vi "mainVI.vi"() -> ()   [LabVIEW 2019]
panel:
  out "Waveform Graph":dbl[][](graph)
  in  "New plot":bool
  in  "stop":bool
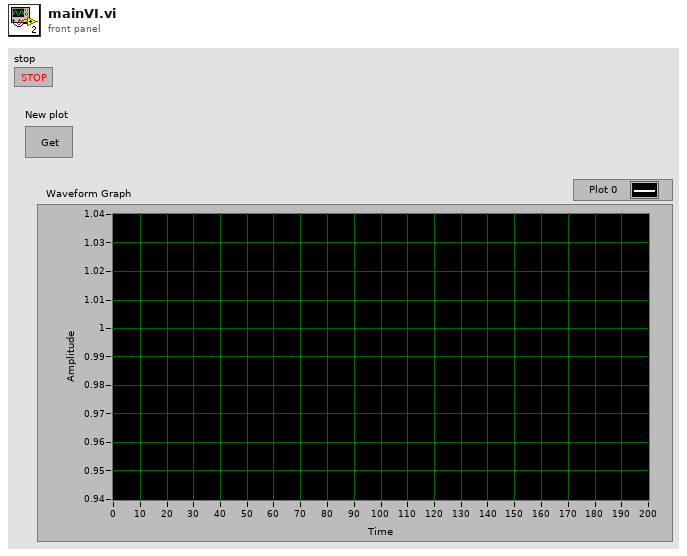
[diagram p1: front panel]
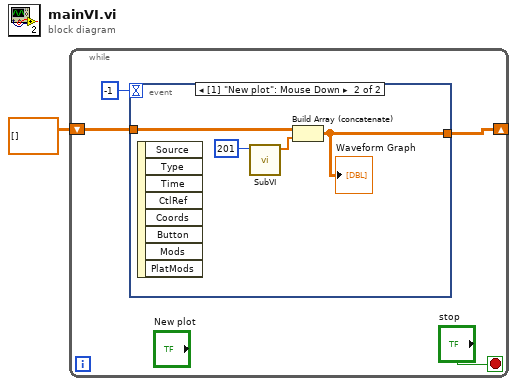
[diagram p0: block diagram]
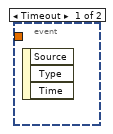
[diagram p2: hidden frame]
diagram:
  n1 = while {
    shift-right: [w3] -> _
    shift-left: dbl[][] [] -> [w2]
    stop <- "stop" stop-if-true
    n2 = event shown="[1] \"New plot\": Mouse Down" {
      selector: _ -> [_ _]
      dyn-events: _ -> [_ _]
      timeout: -1 -> [_ _]
      tunnel: [_ w7] -> w3
      tunnel: w2 -> [_ w6]
      event Timeout {
        n3 = event-data() -> ()  [unwired: 1 in, 3 out]
      }
      event "New plot": Mouse Down {
        n4 = event-data() -> ()  [unwired: 1 in, 8 out]
        n5 = call "SubVI.vi"("Points"=201) -> ("Disorder Pattern 2"=w8:dbl[])  [unwired: 8 in]
        n6 = Build Array (concatenate)(w6, w8) -> (w7:dbl[][])
        "Waveform Graph" <- w7
      }
    }
  }
